vi "Wizard Read Database.vi"(2 "error in (no error)":errorcluster, 3 "Database Location":path) -> (0 "error out":errorcluster, 1 "Database":string[][](array[string]))   [LabVIEW 2014]
uses:
  <vilib>/addons/_office/excel.llb/Excel Get Data ([str]).vi
  <vilib>/Utility/NIReport.llb/NI_report.lvclass
  <vilib>/addons/_office/NI_ReportGenerationToolkit.lvlib
  <vilib>/Utility/NIReport.llb/Excel/NI_Excel.lvclass
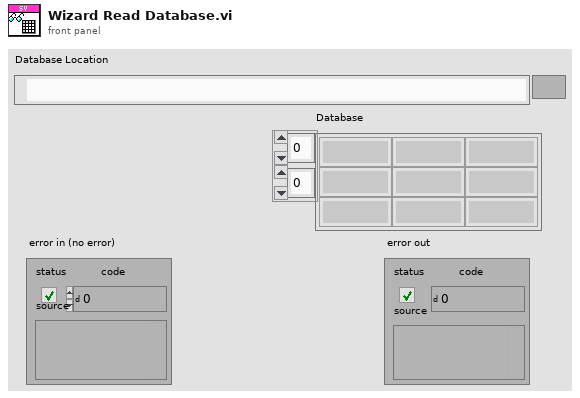
[diagram p1: front panel]
types:
  T1 = enum16{"maximized", "minimized", "normal", "no change"}
  T2 = enum16{"Standard Report", "HTML", "Word", "Excel"}
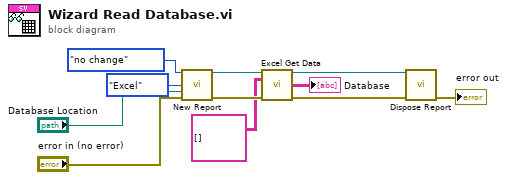
[diagram p0: block diagram]
diagram:
  n1 = call <vilib>:"New Report.vi"("window state (normal)"=T1."no change", "report type"=T2."Excel", "template (empty)"="Database Location", "error in (no error)"="error in (no error)") -> ("report out"=w7:refnum<class "NI_report.lvclass">, "error out"=w6:errorcluster)  [unwired: 10 in]
  n2 = call-poly <vilib>:"Excel Get Data.vi"("report in"=w7, "data type"=string[][] [], "error in (no error)"=w6) -> ("report out"=w3:refnum<class "NI_report.lvclass">, "data"=→"Database":string[][], "error out"=w2:errorcluster)  [unwired: 10 in]
  n3 = call-dynamic "Dispose Report.vi"("report in"=w3, "error in (no error)"=w2) -> ("error out"=→"error out":errorcluster)  [unwired: 13 in]
